vi "Menu - Toggle Checked State.vi"(8 "error in (no error)":errorcluster, 10 "item tag":string, 11 "menu reference":refnum<k9>) -> (0 "error out":errorcluster)   [LabVIEW 2015]
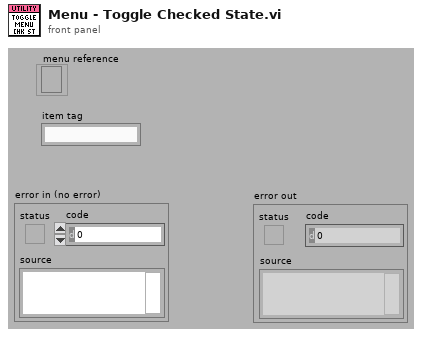
[diagram p1: front panel]
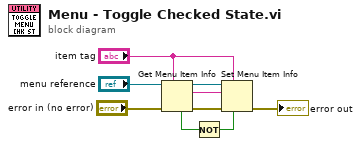
[diagram p0: block diagram]
diagram:
  n1 = Get Menu Item Info(7:"item tag", 8:"error in (no error)", 11:"menu reference") -> (0:w2:errorcluster, 2:w8:string, 3:w9:refnum<k9>, 4:w7:bool)  [unwired: 3 out]
  n2 = Not(x=w7) -> (.not. x?=w6:bool)
  n3 = Set Menu Item Info(6:w6, 7:"item tag", 8:w2, 10:w8, 11:w9) -> (0:→"error out":errorcluster)  [unwired: 3 out]
